vi "Intake Pneumatic.vi"(11 "Operator A Button":bool) -> ()   [LabVIEW 2019]
uses:
  .Team Code/Robot Global Data.vi
  <vilib>/Rock Robotics/WPI/Solenoid/WPI_SolenoidValue.ctl
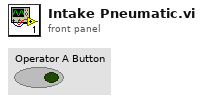
[diagram p1: front panel]
types:
  T1 = typedef "WPI_SolenoidValue.ctl" = enum16{"Off", "On", "Forward", "Reverse"}
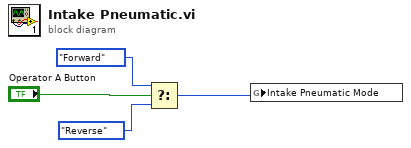
[diagram p0: block diagram]
diagram:
  n1 = Select(t=WPI_SolenoidValue."Forward" ("Value"), s="Operator A Button", f=WPI_SolenoidValue."Reverse" ("Value")) -> (s? t:f=w1:T1)
  n2 = global write "Robot Global Data.vi" "Intake Pneumatic Mode"(w1) -> ()
